vi "Location to Insecure Address.vi"(11 "Location":T1) -> (3 "String":string)   [LabVIEW 2021, in "Measurement Service Helpers.lvlib"]
uses:
  Measurement Service Helpers.lvlib
  <vilib>/MeasurementLink/MeasurementLink Discovery Client/RPC Messages/ni_measurementlink_discovery_v1_ServiceLocation.ctl
  <vilib>/MeasurementLink/MeasurementLink Discovery Client/MeasurementLink Discovery Client.lvlib
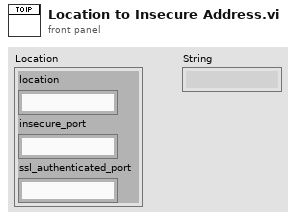
[diagram p1: front panel]
types:
  T1 = typedef "MeasurementLink Discovery Client.lvlib/ni_measurementlink_discovery_v1_ServiceLocation.ctl" = cluster{"location":string, "insecure_port":string, "ssl_authenticated_port":string}
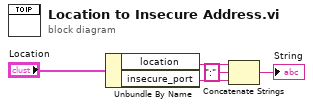
[diagram p0: block diagram]
diagram:
  n1 = Unbundle By Name("Location") -> ("location"=w2:string, "insecure_port"=w3:string)
  n2 = Concatenate Strings(w2, ":" ("string"), w3) -> (→"String":string)
